vi "QuickDrop Set As Main VI.vi"(6 "Variant in":variant, 7 "Shift Pressed?":bool, 8 "error in (no error)":errorcluster, 10 "QD Combo Box Ref":refnum<vi>, 11 "QD Launch VI Ref":refnum<vi>) -> (0 "error out":errorcluster, 4 "Variant out":variant)   [LabVIEW 2016]
doc: "Show the front panel of the top level referenced in the project description.\n\nDefault Shortcut - [$]"
panel:
  in  "Undo Name":string="Quick Drop Keyboard Shortcut"
  # "Specify the name of the Undo transaction"
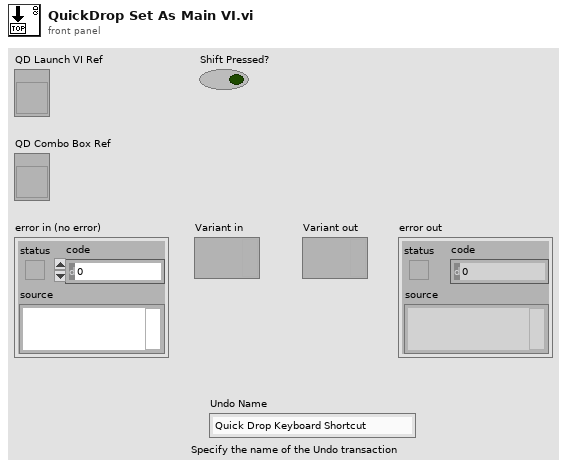
[diagram p1: front panel]
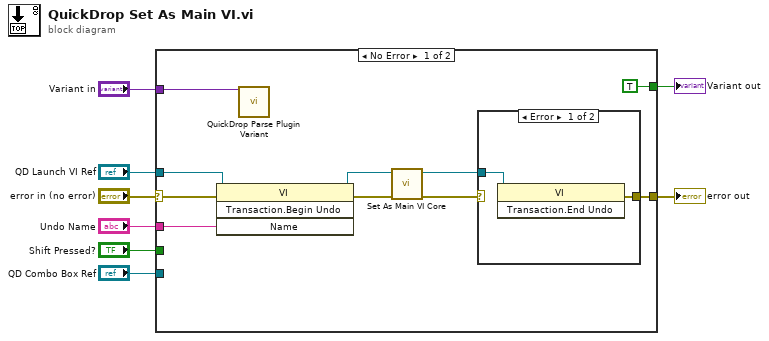
[diagram p0: block diagram]
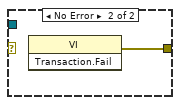
[diagram p2: hidden frame]
diagram:
  n1 = case shown="No Error" "error in (no error)" {
    selector: "error in (no error)" -> [w17 w22]
    tunnel: [w13 w22] -> w7
    tunnel: "QD Launch VI Ref" -> [w16 _]
    tunnel: "Shift Pressed?" -> [_ _]
    tunnel: "QD Combo Box Ref" -> [_ _]
    tunnel: "Variant in" -> [w18 _]
    tunnel: "Undo Name" -> [w15 _]
    tunnel: [TRUE _] -> w1
    frame No Error {
      n2 = invoke class="VI" method="Transaction.Begin Undo"(reference=w16, error in=w17, "Name"=w15) -> (reference out=w11:refnum<vi>, error out=w12:errorcluster)  [unwired: 1 in, 2 out]
      n3 = call <vilib>:"QuickDrop Parse Plugin Variant.vi"("QDKS Variant in"=w18) -> ()  [unwired: 12 in, 3 out]
      n4 = call "Set As Main VI Core.vi"("error in (no error)"=w12, "Calling VI Ref in"=w11) -> ("error out"=w10:errorcluster, "Calling VI Ref out"=w9:refnum<vi>)  [unwired: 8 in]
      n5 = case shown="Error" w10 {
        tunnel: [w20 w21] -> w13
        tunnel: w9 -> [w19 _]
        frame Error {
          n6 = invoke class="VI" method="Transaction.End Undo"(reference=w19) -> (error out=w20:errorcluster)  [unwired: 2 in, 2 out]
        }
        frame No Error {
          n7 = invoke class="VI" method="Transaction.Fail"() -> (error out=w21:errorcluster)  [unwired: 3 in, 2 out]
        }
      }
    }
    frame Error {
    }
  }
  "error out" <- w7
  "Variant out" <- w1
